vi "StateToColor.vi"(8 "error in (no error)":errorcluster, 11 "Flags in":refnum<class "Flags.lvclass">) -> (0 "error out":errorcluster, 2 "RoomNumFlags":T1={"Flag State"=[1, 3, 5, 7]}, 3 "Flags out":refnum<class "Flags.lvclass">)   [LabVIEW 2015, in "Flags.lvclass"]
uses:
  Flags.lvclass
  ColorFlags.ctl
  Flags.lvclass/Flags.ctl
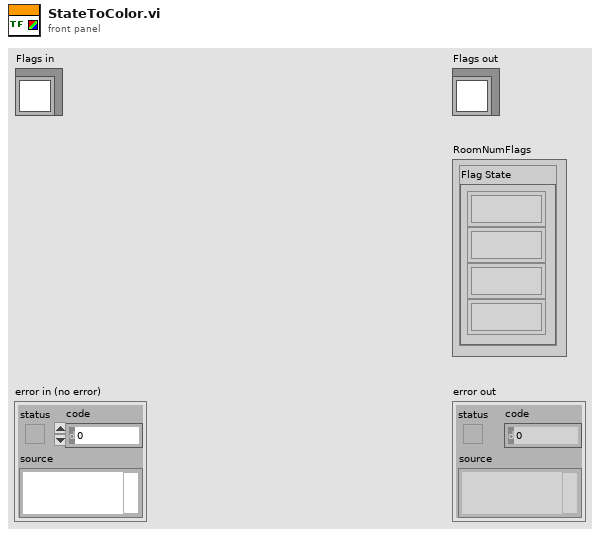
[diagram p1: front panel]
types:
  T1 = typedef "Flags.lvclass/ColorFlags.ctl" = cluster{"Flag State":u8[]}
  T2 = typedef "Flags.lvclass/ColorEnum.ctl" = enum8{"Red", "Blue", "Green", "Yellow"}
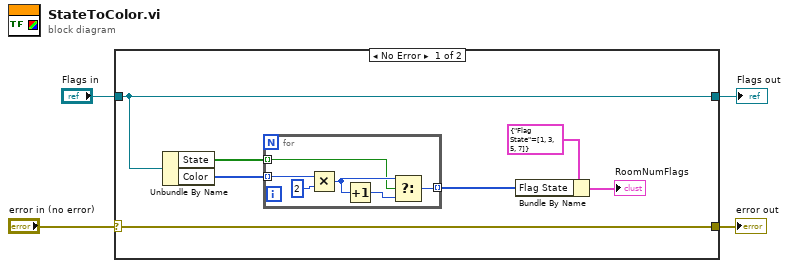
[diagram p0: block diagram]
diagram:
  n1 = case shown="No Error" "error in (no error)" {
    selector: "error in (no error)" -> [w11 w19]
    tunnel: [w11 w19] -> w3
    tunnel: [w10 w18] -> w1
    tunnel: "Flags in" -> [w10 w18]
    frame No Error {
      n2 = Unbundle By Name(w10) -> ("State"=w5:bool[], "Color"=w9:T2[])
      n3 = for {
        tunnel: w9 -> [w16] mode=indexing
        tunnel: [w13] -> w6 mode=indexing
        tunnel: w5 -> [w12] mode=indexing
        n4 = Multiply(x=w16, y=u8 2) -> (x*y=w14:u8)
        n5 = Increment(x=w14) -> (x+1=w15:u8)
        n6 = Select(t=w14, s=w12, f=w15) -> (s? t:f=w13:u8)
      }
      n7 = Bundle By Name(cluster=T1 {"Flag State"=[1, 3, 5, 7]} ("Array"), "Flag State"=w6) -> (→"RoomNumFlags":T1)
    }
    frame Error {
    }
  }
  "error out" <- w3
  "Flags out" <- w1
